vi "snap.vi"(4 "error in (no error)":errorcluster, 6 "y":i32, 7 "x":i32) -> (0 "error out 2":errorcluster, 1 "ImgCnt":i32, 2 "Valid":bool, 3 "Image":i32[][](graph))   [LabVIEW 2012]
panel:
  out "first":u32
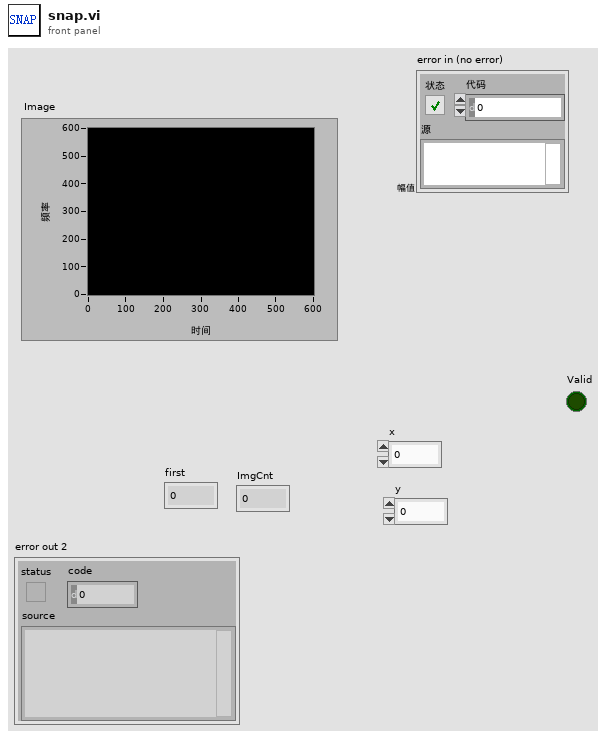
[diagram p1: front panel]
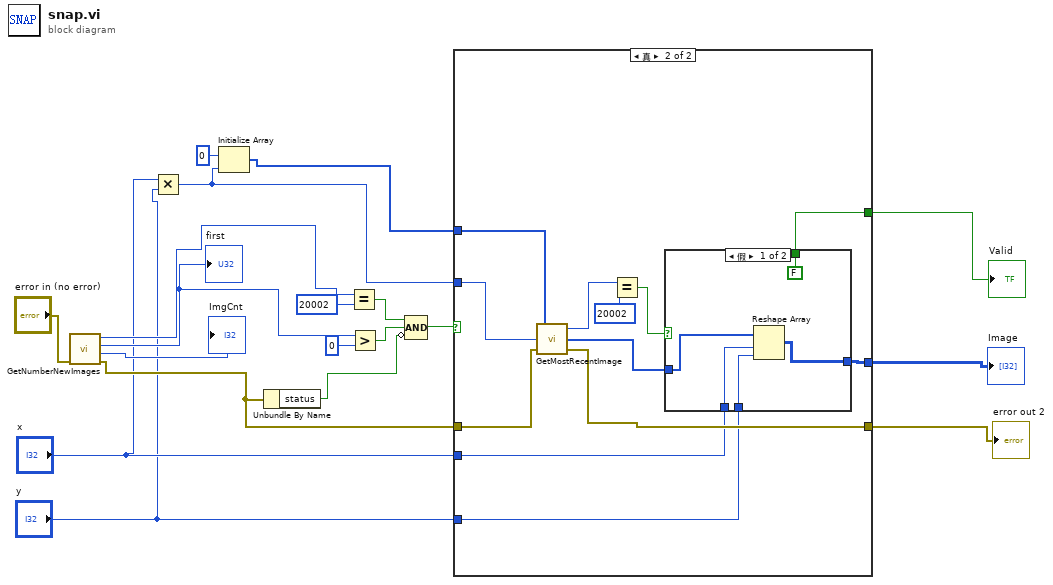
[diagram p0: block diagram]
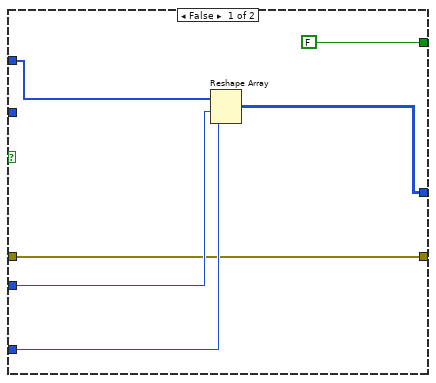
[diagram p2: hidden frame]
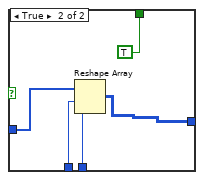
[diagram p3: hidden frame]
diagram:
  n1 = call <userlib>:"GetNumberNewImages.vi"("error in (no error)"="error in (no error)") -> ("error out"=w9:errorcluster, "last"=→"ImgCnt":i32, "first"=w16:u32, "DLL error code"=w10:u32)  [unwired: 3 in]
  "first" <- w16
  n2 = Multiply(x="x", y="y") -> (x*y=w1:i32)
  n3 = Initialize Array(i16 0 ("元素"), w1) -> (w5:i16[])
  n4 = Unbundle By Name(w9) -> ("status"=w12:bool)
  n5 = Equal?(x=w10, y=u32 20002) -> (x = y?=w14:bool)
  n6 = Greater?(x=w16, y=u32 0) -> (0:w13:bool)
  n7 = Compound Arithmetic op=AND(w14, w13, invert w12) -> (w11:bool)
  n8 = case shown="真" w11 {
    tunnel: w9 -> [w20 w33]
    tunnel: [w20 w32] -> w8
    tunnel: w5 -> [w25 w31]
    tunnel: [w22 w30] -> w7
    tunnel: "x" -> [w24 w29]
    tunnel: "y" -> [w23 w28]
    tunnel: [FALSE ("Valid") w27] -> w6
    tunnel: w1 -> [_ w26]
    frame False {
      n9 = Reshape Array(w25, w24, w23) -> (w22:i16[][])
    }
    frame True {
      n10 = call <userlib>:"GetMostRecentImage.vi"("error in (no error)"=w33, "size"=w26, "array"=w31) -> ("error out"=w32:errorcluster, "array"=w36:i32[], "DLL error code"=w34:u32)
      n11 = Equal?(x=w34, y=u32 20002) -> (x = y?=w35:bool)
      n12 = case shown="假" w35 {
        tunnel: w36 -> [w41 w47]
        tunnel: [w38 w46] -> w30
        tunnel: w29 -> [w40 w45]
        tunnel: w28 -> [w39 w44]
        tunnel: [FALSE ("Valid") TRUE ("Valid")] -> w27
        frame False {
          n13 = Reshape Array(w41, w40, w39) -> (w38:i32[][])
        }
        frame True {
          n14 = Reshape Array(w47, w45, w44) -> (w46:i32[][])
        }
      }
    }
  }
  "error out 2" <- w8
  "Image" <- w7
  "Valid" <- w6
